vi "Write ref.vi"(8 "error in":errorcluster, 10 "ref":refnum<vi>, 11 "stats in":refnum<class "stats.lvclass">) -> (0 "error out":errorcluster, 3 "stats out":refnum<class "stats.lvclass">)   [LabVIEW 2016, in "stats.lvclass"]
uses:
  stats.lvclass
  stats.lvclass/stats.ctl
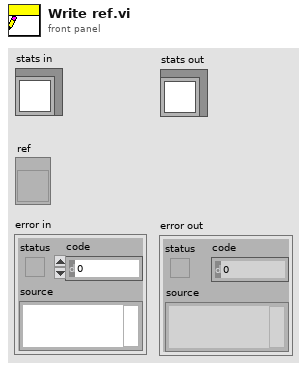
[diagram p1: front panel]
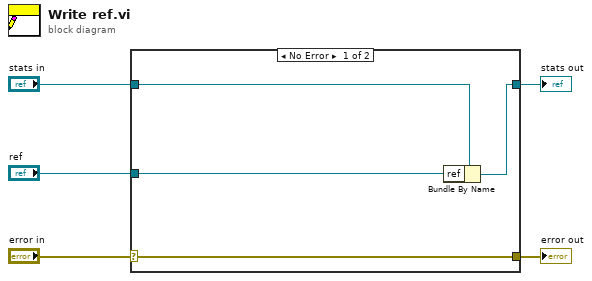
[diagram p0: block diagram]
diagram:
  n1 = case shown="No Error" "error in" {
    selector: "error in" -> [w9 w10]
    tunnel: [w9 w10] -> w4
    tunnel: [w7 w11] -> w2
    tunnel: "stats in" -> [w8 w11]
    tunnel: "ref" -> [w6 _]
    frame No Error {
      n2 = Bundle By Name(cluster=w8, "ref"=w6) -> (w7:refnum<class "stats.lvclass">)
    }
    frame Error {
    }
  }
  "error out" <- w4
  "stats out" <- w2
